vi "Create All Message Queues.vi"(8 "error in (no error)":cluster{"状态":bool, "代码":i32, "源":string} caption="错误输入（无错误）") -> (0 "error out":cluster{"状态":bool, "代码":i32, "源":string} caption="错误输出", 3 "消息队列输出":T1)   [LabVIEW 2015, in "Message Queue.lvlib"]
doc: "本VI用于创建应用程序所需的所有消息队列。如应用程序需要两个以上消息队列，可右键单击上面的“消息队列”常量并选择打开自定义类型，将新的消息队列添加至该自定义类型，然后通过本VI进行初始化。"
uses:
  Message Queue.lvlib
  All Message Queues.ctl
  Message Cluster.ctl
  Enqueue Message (Single).vi
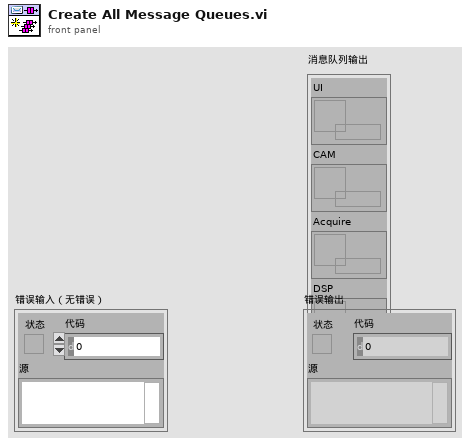
[diagram p1: front panel]
types:
  T1 = typedef "Message Queue.lvlib/All Message Queues.ctl" = cluster{"UI":refnum<queue>, "CAM":refnum<queue>, "Acquire":refnum<queue>, "DSP":refnum<queue>}
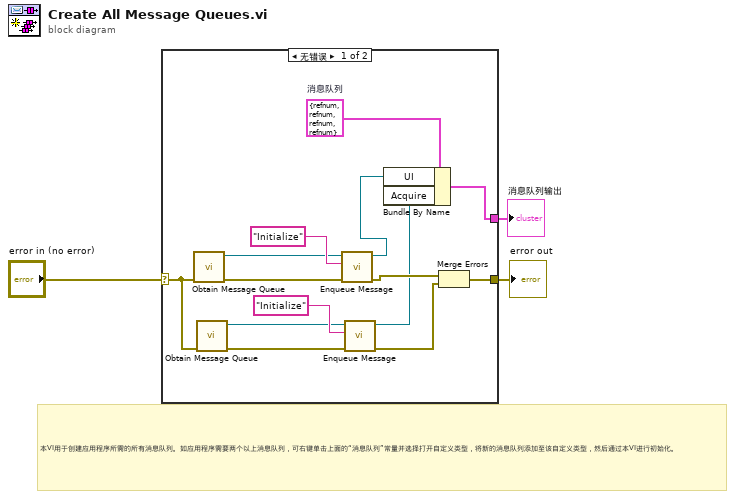
[diagram p0: block diagram]
diagram:
  # "本VI用于创建应用程序所需的所有消息队列。如应用程序需要两个以上消息队列，可右键单击上面的“消息队列”常量并选择打开自定义类型，将新的消息队列添加至该自定义类型，然后通过本VI进行初始化。"
  n1 = case shown="无错误" "error in (no error)" {
    selector: "error in (no error)" -> [w9 w18]
    tunnel: [w8 w18] -> w3
    tunnel: [w16 _] -> w2
    frame No Error {
      w17 = T1 {"UI"=refnum, "CAM"=refnum, "Acquire"=refnum, "DSP"=refnum}  # 消息队列
      n2 = call "Obtain Message Queue.vi"("error in (no error)"=w9) -> ("error out"=w15:cluster{"状态":bool, "代码":i32, "源":string}, "消息队列"=w13:refnum<queue>)  [unwired: 9 in]
      n3 = call "Obtain Message Queue.vi"("error in (no error)"=w9) -> ("error out"=w12:cluster{"状态":bool, "代码":i32, "源":string}, "消息队列"=w10:refnum<queue>)  [unwired: 9 in]
      n4 = call-poly "Enqueue Message.vi"("error in (no error)"=w15, "消息"="Initialize" ("Message"), "消息队列"=w13) -> ("error out"=w7:cluster{"状态":bool, "代码":i32, "源":string}, "消息队列副本"=w4:refnum<queue>)  [unwired: 7 in]
      n5 = call-poly "Enqueue Message.vi"("error in (no error)"=w12, "消息"="Initialize" ("Message"), "消息队列"=w10) -> ("error out"=w6:cluster{"状态":bool, "代码":i32, "源":string}, "消息队列副本"=w5:refnum<queue>)  [unwired: 7 in]
      n6 = Bundle By Name(cluster=w17, "UI"=w4, "Acquire"=w5) -> (w16:T1)
      n7 = Merge Errors(w7, w6) -> (w8:errorcluster)
    }
    frame Error {
    }
  }
  "消息队列输出" <- w2
  "error out" <- w3
